vi "DVFS.vi"(1 "Start string":string, 2 "string":string, 4 "end string":string) -> (6 "Output":i32[](array[numeric]), 7 "size(s)":i32, 8 "invalid data output":bool)   [LabVIEW 2018]
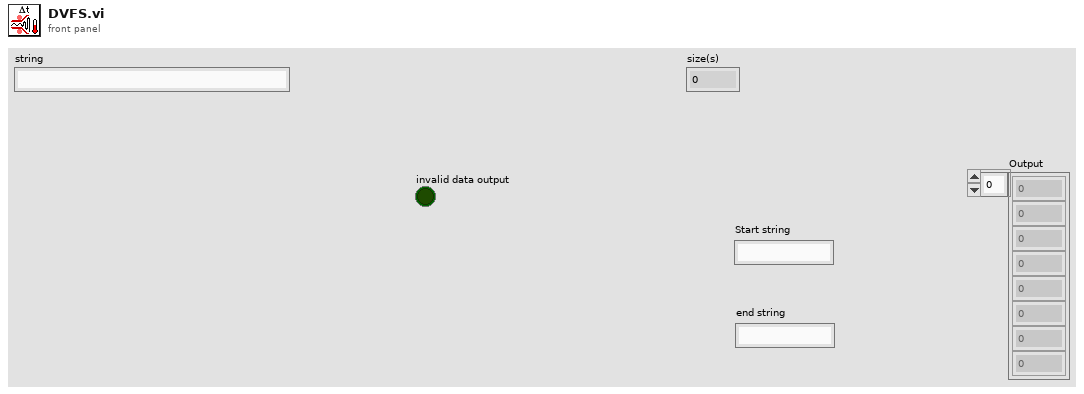
[diagram p1: front panel]
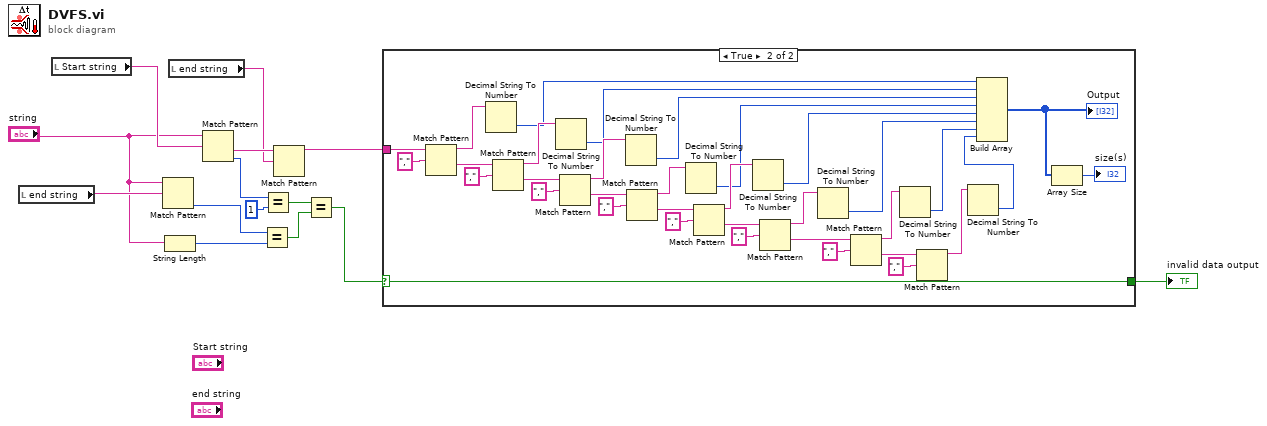
[diagram p0: block diagram]
diagram:
  n1 = local read "end string"() -> (w3:string)
  n2 = local read "Start string"() -> (w4:string)
  n3 = Match Pattern(string="string", regular expression=w3) -> (offset past match=w12:i32)  [unwired: 1 in, 3 out]
  n4 = String Length(string="string") -> (length=w11:i32)
  n5 = local read "end string"() -> (w2:string)
  n6 = Match Pattern(string="string", regular expression=w4) -> (after substring=w5:string, offset past match=w14:i32)  [unwired: 1 in, 2 out]
  n7 = Equal?(x=w12, y=w11) -> (x = y?=w9:bool)
  n8 = Equal?(x=w14, y=1) -> (x = y?=w10:bool)
  n9 = Match Pattern(string=w5, regular expression=w2) -> (before substring=w6:string)  [unwired: 1 in, 3 out]
  n10 = Equal?(x=w10, y=w9) -> (x = y?=w8:bool)
  n11 = case shown="True" w8 {
    selector: w8 -> [w15 w49]
    tunnel: [w15 w49] -> w7
    tunnel: w6 -> [_ w48]
    frame False {
    }
    frame True {
      n12 = Match Pattern(string=w48, regular expression=",") -> (before substring=w33:string, after substring=w47:string)  [unwired: 1 in, 2 out]
      n13 = Decimal String To Number(string=w33) -> (number=w18:i32)  [unwired: 2 in, 1 out]
      n14 = Match Pattern(string=w47, regular expression=",") -> (before substring=w32:string, after substring=w45:string)  [unwired: 1 in, 2 out]
      n15 = Decimal String To Number(string=w32) -> (number=w19:i32)  [unwired: 2 in, 1 out]
      n16 = Match Pattern(string=w45, regular expression=",") -> (before substring=w31:string, after substring=w43:string)  [unwired: 1 in, 2 out]
      n17 = Decimal String To Number(string=w31) -> (number=w20:i32)  [unwired: 2 in, 1 out]
      n18 = Match Pattern(string=w43, regular expression=",") -> (before substring=w30:string, after substring=w41:string)  [unwired: 1 in, 2 out]
      n19 = Decimal String To Number(string=w30) -> (number=w21:i32)  [unwired: 2 in, 1 out]
      n20 = Match Pattern(string=w41, regular expression=",") -> (before substring=w29:string, after substring=w39:string)  [unwired: 1 in, 2 out]
      n21 = Decimal String To Number(string=w29) -> (number=w22:i32)  [unwired: 2 in, 1 out]
      n22 = Match Pattern(string=w39, regular expression=",") -> (before substring=w28:string, after substring=w37:string)  [unwired: 1 in, 2 out]
      n23 = Decimal String To Number(string=w28) -> (number=w23:i32)  [unwired: 2 in, 1 out]
      n24 = Match Pattern(string=w37, regular expression=",") -> (before substring=w27:string, after substring=w35:string)  [unwired: 1 in, 2 out]
      n25 = Decimal String To Number(string=w27) -> (number=w24:i32)  [unwired: 2 in, 1 out]
      n26 = Match Pattern(string=w35, regular expression=",") -> (before substring=w26:string)  [unwired: 1 in, 3 out]
      n27 = Decimal String To Number(string=w26) -> (number=w25:i32)  [unwired: 2 in, 1 out]
      n28 = Build Array(w18, w19, w20, w21, w22, w23, w24, w25) -> (w16:i32[])
      "Output" <- w16
      n29 = Array Size(array=w16) -> (size(s)=→"size(s)":i32)
    }
  }
  "invalid data output" <- w7
